vi "DefenderChute.vi"(6 "Current State":dbl=1.0, 7 "IA State Input 2":T1, 9 "balls":T5[](array[typedef])=[{"x"=-974.5169677734375, "y"=-3444.3310546875, "timestamp"=timestamp(2082759045.994995 s since 1904-01-01), "Vel_x"=0.0, "Vel_y"=0.0}], 10 "Field Size in":T6={"line_width"=10, "field_length"=9000, "field_width"=6000, "boundary_width"=250, "referee_width"=425, "goal_width"=700, "goal_depth"=180, "goal_wall_width"=20, "center_circle_radius"=500, "defense_radius"=500, "defense_stretch"=350, "free_kick_from_defense_dist"=700, "penalty_spot_from_field_line_dist"=450, "penalty_line_from_spot_dist"=350}, 11 "Robot in":T2={"id"=5, "function"=enum."Attacker", "x"=-983.1382446289062, "y"=-3000.010498046875, "orientation"=-1.5516623258590698, "v_tangent"=0.0, "v_normal"=0.0, "v_ang"=0.0, "kick_x"=0.0, "kick_z"=0.0, "dribble"=FALSE, "Timestamp"=timestamp(2082759045.994995 s since 1904-01-01), "dest_x"=0.0, "dest_y"=0.0, "dest_orientation"=0.0, "estimatives"={"est_v_tangent"=0.0, "est_v_normal"=0.0, "est_vx"=0.0, "est_vy"=0.0}, "dest_x_kick"=0.0, "dest_y_kick"=0.0, "Gap Coord"=[], "States"=enum."GoToTangent"}) -> (1 "Next State":dbl=1.0, 3 "Robot out":T2={"id"=5, "function"=enum."Attacker", "x"=-983.1382446289062, "y"=-3000.010498046875, "orientation"=-1.5516623258590698, "v_tangent"=0.0001540345015520423, "v_normal"=0.008599927144915481, "v_ang"=0.002668461263266586, "kick_x"=0.0, "kick_z"=0.0, "dribble"=FALSE, "Timestamp"=timestamp(2082759045.994995 s since 1904-01-01), "dest_x"=0.0, "dest_y"=0.0, "dest_orientation"=0.0, "estimatives"={"est_v_tangent"=0.0, "est_v_normal"=0.0, "est_vx"=0.0, "est_vy"=0.0}, "dest_x_kick"=0.0, "dest_y_kick"=0.0, "Gap Coord"=[], "States"=enum."GoToTangent"})   [LabVIEW 2016]
uses:
  Core/AI Robot.ctl
  Functions Enum.ctl
  AttackerStates.ctl
  Core/Field Size.ctl
  Core/AI Ball.ctl
  Core/AI Input.ctl
  Core/AI Judge.ctl
  Command Enum.ctl
  <vilib>/Analysis/coordinate.llb/2D Cartesian Coordinate Rotation (Scalar).vi
  <vilib>/Analysis/NI_AALPro.lvlib
panel:
  in  "Dist a frente da bola 2":dbl=150.0 format="%#_13g"
  in  "reckon timer":dbl=1.0 caption="Time Target (s)"
  out "Elapsed Time (s) 2":dbl caption="Elapsed Time (s)"
  out "Waveform Chart":dbl(graph)
  out "Elapsed Time (s)":dbl
  in  "Time Target \nto transition":dbl=0.5 caption="Time Target (s)"
  in  "Longe":dbl=300.0 format="%#_13g"
  in  "Cone de chute":dbl=0.09 format="%#_13g"
  in  "Perto":dbl=300.0 format="%#_13g"
  in  "Cone de rotação":dbl=1.1 format="%#_13g"
  in  "attacker farback":dbl=1500.0 format="%#_13g"
  in  "min dist to kick":dbl=150.0 format="%#_13g"
  in  "Dist a frente da bola":dbl format="%#_13g"
  in  "Constante do Renault":dbl=0.05
  in  "raio da circunferencia":dbl=175.0 format="%#_13g"
  in  "distance between ball and robot":dbl=275.0 format="%#_13g"
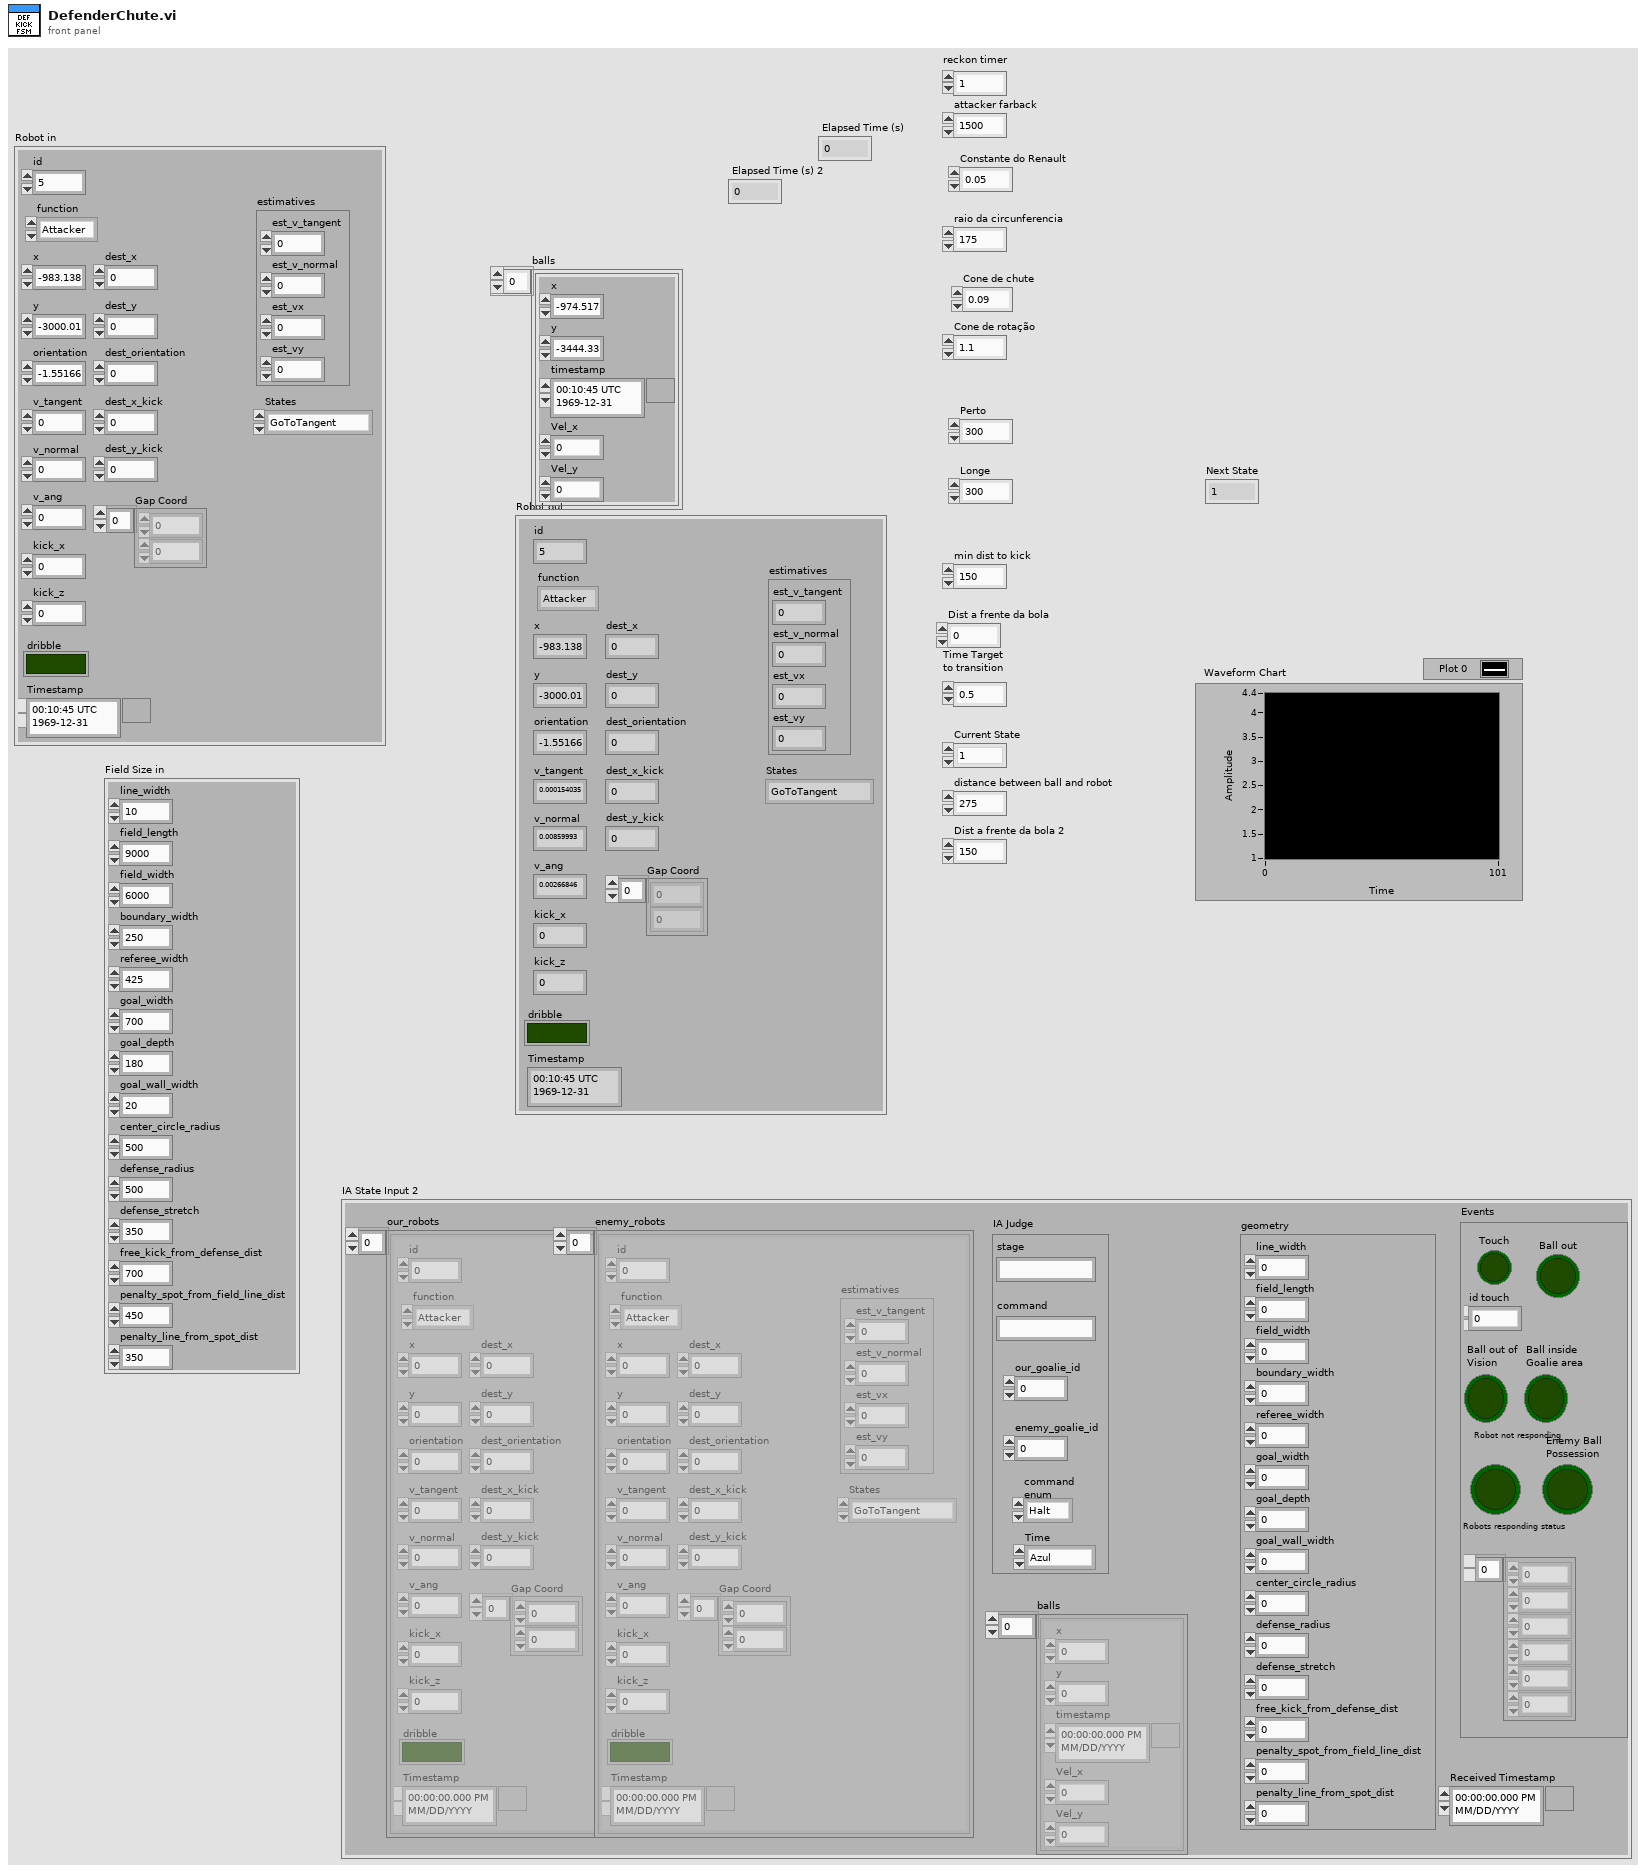
[diagram p1: front panel]
types:
  T1 = typedef "AI Input.ctl" = cluster{"our_robots":T2[], "enemy_robots":T2[], "balls":T5[], "geometry":T6, "IA Judge":T7, "Received Timestamp":timestamp, "Events":cluster{"Touch":bool, "Ball out":bool, "id touch":dbl, "Ball out of \nVision":bool, "Ball inside \nGoalie area":bool, "Robot not responding":bool, "Robots responding status":dbl[], "Enemy Ball \nPossession":bool}}
  T2 = typedef "AI Robot.ctl" = cluster{"id":u32, "function":T3, "x":dbl, "y":dbl, "orientation":dbl, "v_tangent":dbl, "v_normal":dbl, "v_ang":dbl, "kick_x":dbl, "kick_z":dbl, "dribble":bool, "Timestamp":timestamp, "dest_x":dbl, "dest_y":dbl, "dest_orientation":dbl, "estimatives":cluster{"est_v_tangent":dbl, "est_v_normal":dbl, "est_vx":dbl, "est_vy":dbl}, "dest_x_kick":dbl, "dest_y_kick":dbl, "Gap Coord":dbl[], "States":T4}
  T3 = typedef "Functions Enum.ctl" = enum16{"Attacker", "Goalie", "Defender", "Striker", "Goto 0", "Dummy", "Kicker", "ZigZag"}
  T4 = typedef "AttackerStates.ctl" = enum16{"Pass", "GoToTangent", "BallGetting", "GoToKick", ""}
  T5 = typedef "AI Ball.ctl" = cluster{"x":dbl, "y":dbl, "timestamp":timestamp, "Vel_x":dbl, "Vel_y":dbl}
  T6 = typedef "Field Size.ctl" = cluster{"line_width":u32, "field_length":u32, "field_width":u32, "boundary_width":u32, "referee_width":u32, "goal_width":u32, "goal_depth":u32, "goal_wall_width":u32, "center_circle_radius":u32, "defense_radius":u32, "defense_stretch":u32, "free_kick_from_defense_dist":u32, "penalty_spot_from_field_line_dist":u32, "penalty_line_from_spot_dist":u32}
  T7 = typedef "AI Judge.ctl" = cluster{"stage":string, "command":string, "our_goalie_id":dbl, "enemy_goalie_id":dbl, "command\nenum":T8, "Time":enum16{"Azul", "Amarelo"}}
  T8 = typedef "Command Enum.ctl" = enum16{"Halt", "Stop", "Force Start", "PKA Normal Start", "Prepare Kickoff Ally", "PKE Normal Start", "Prepare Kickoff Enemy", "Prepare Penalty Ally", "PPA Normal Start", "Prepare Penalty Enemy", "PPE Normal Start", "Direct Free Enemy", "Direct Free Ally", "Indirect Free Enemy", "Indirect Free Ally", "Timeout Enemy", "Timeout Ally", "Goal Enemy", "Goal Ally", "Ball Placement Enemy", "Ball Placement Ally", "None"}
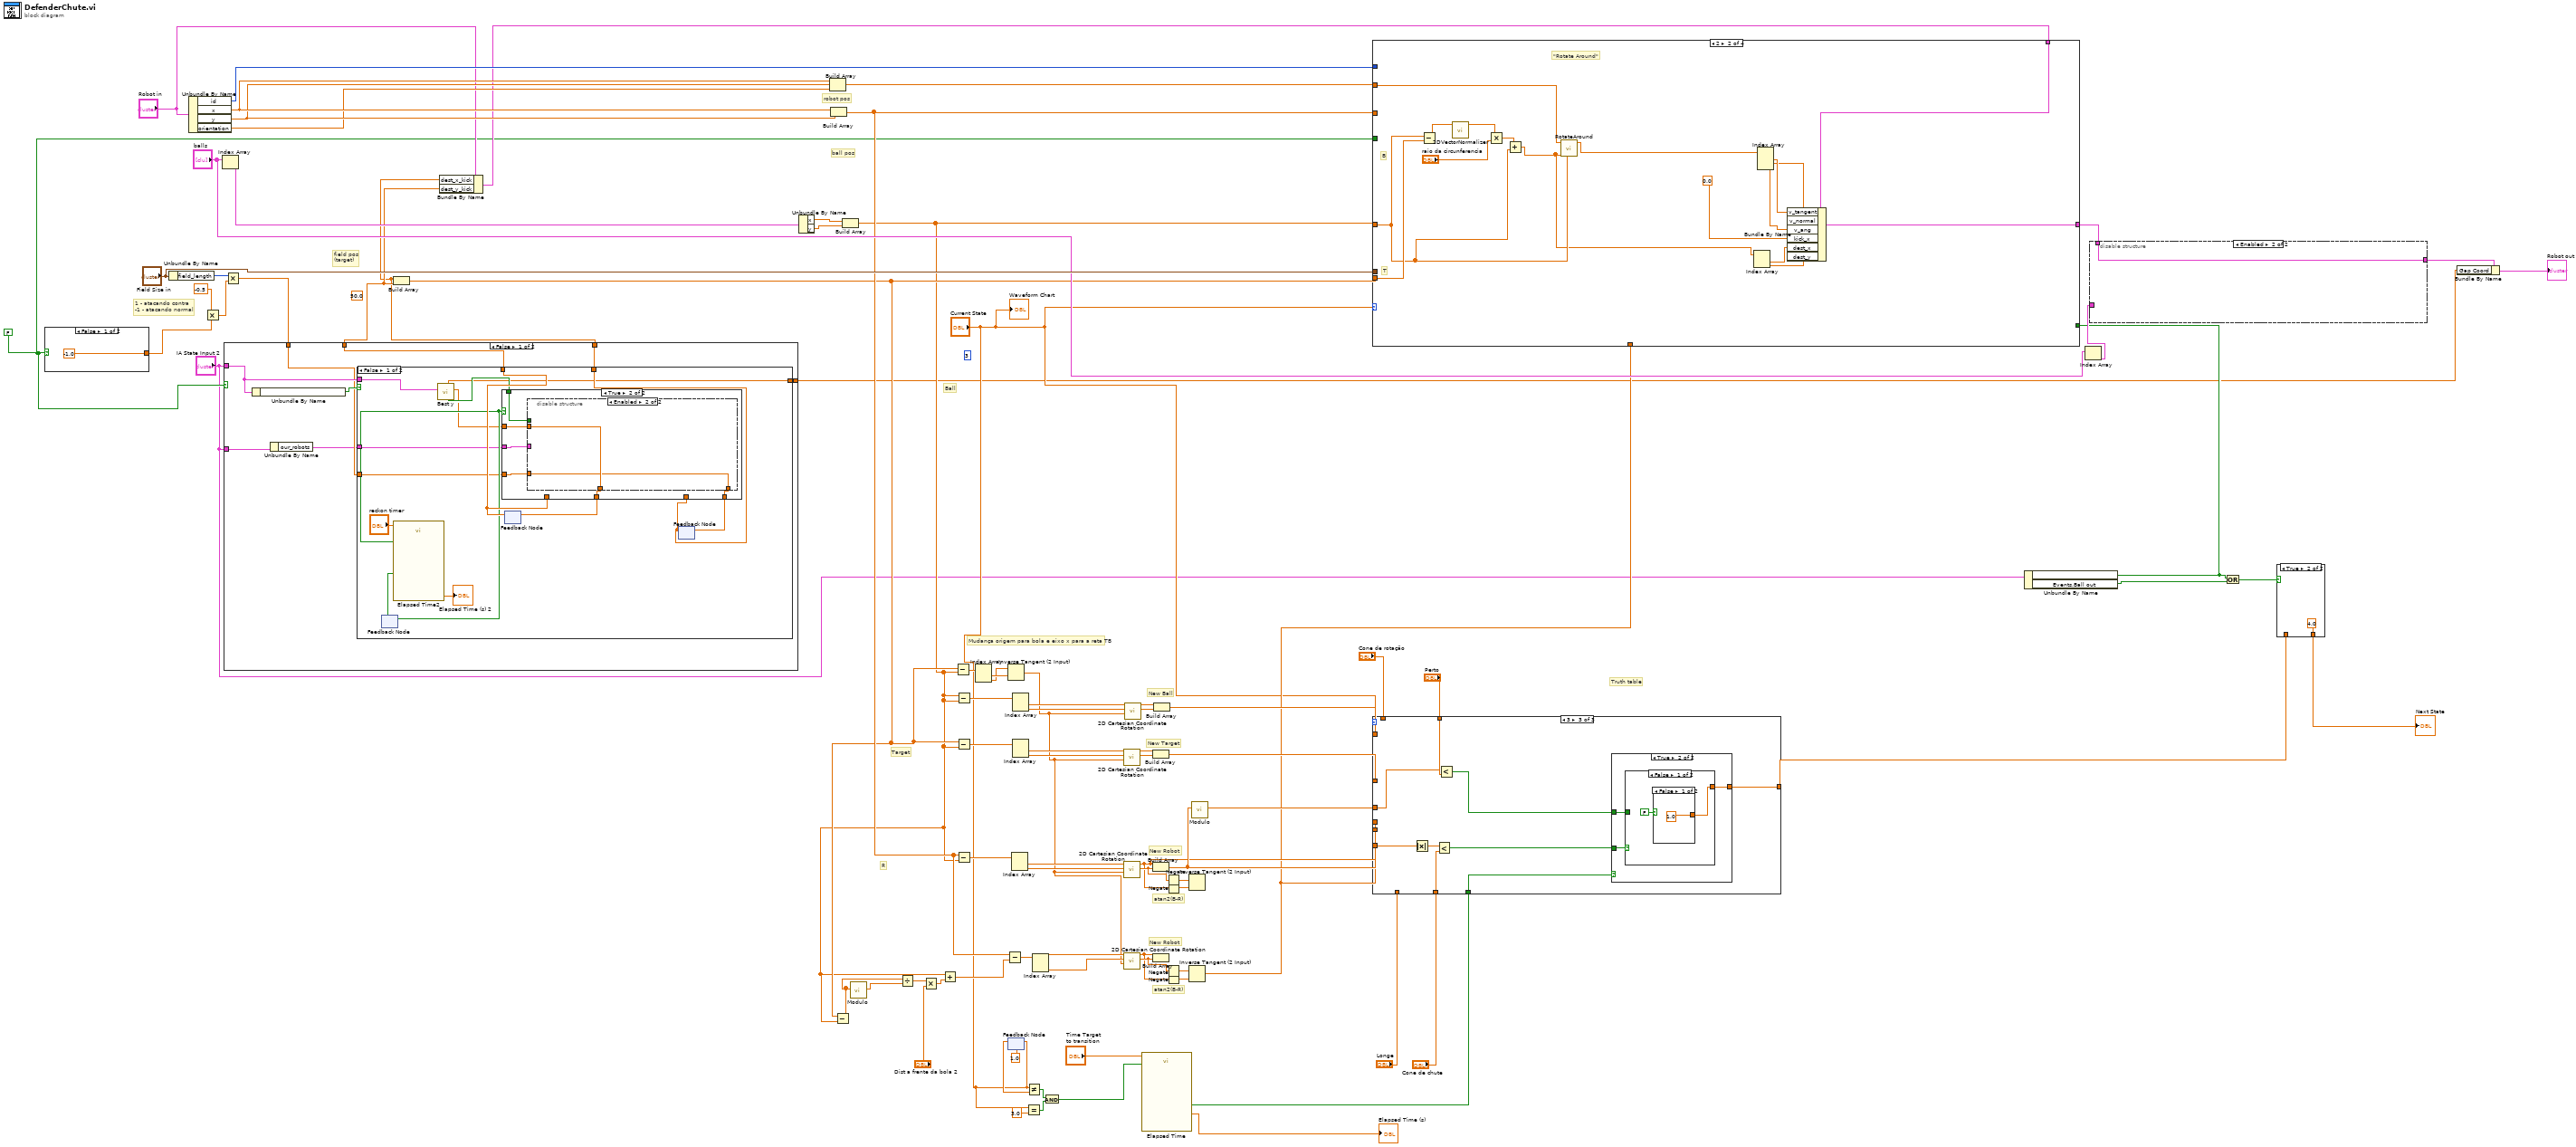
[diagram p0: block diagram]
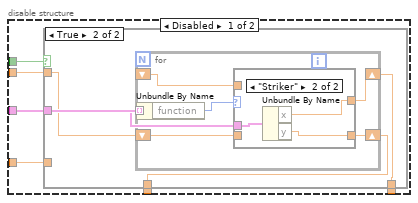
[diagram p3: hidden frame]
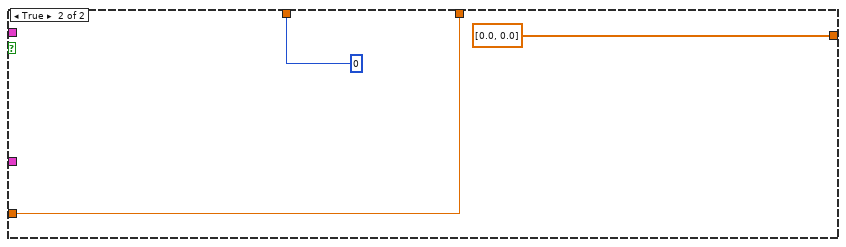
[diagram p6: hidden frame]
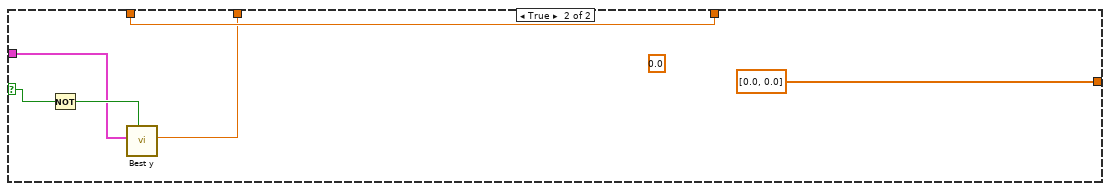
[diagram p7: hidden frame]
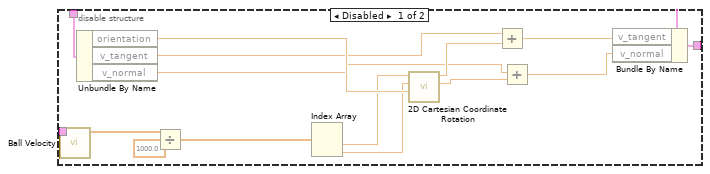
[diagram p8: hidden frame]
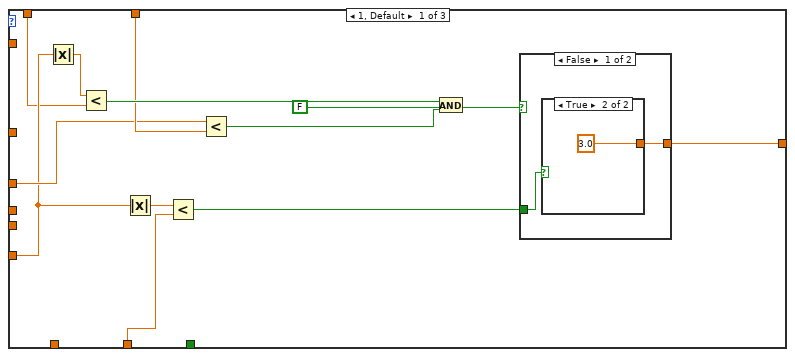
[diagram p9: hidden frame]
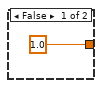
[diagram p10: hidden frame]
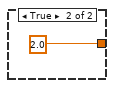
[diagram p11: hidden frame]
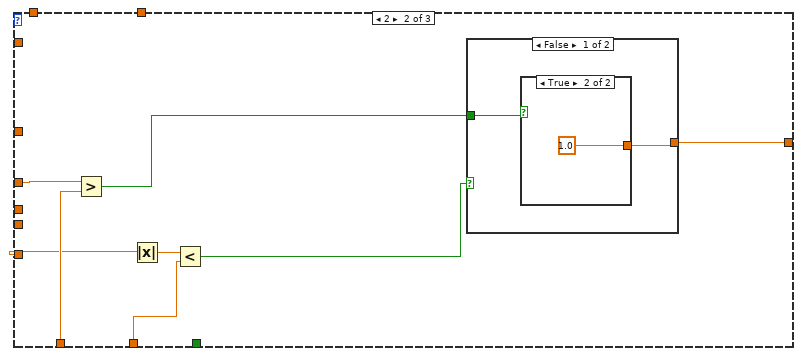
[diagram p12: hidden frame]
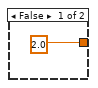
[diagram p13: hidden frame]
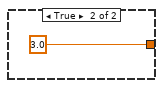
[diagram p14: hidden frame]
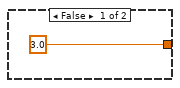
[diagram p15: hidden frame]
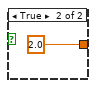
[diagram p16: hidden frame]
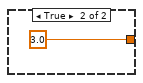
[diagram p17: hidden frame]
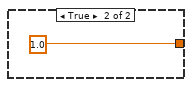
[diagram p19: hidden frame]
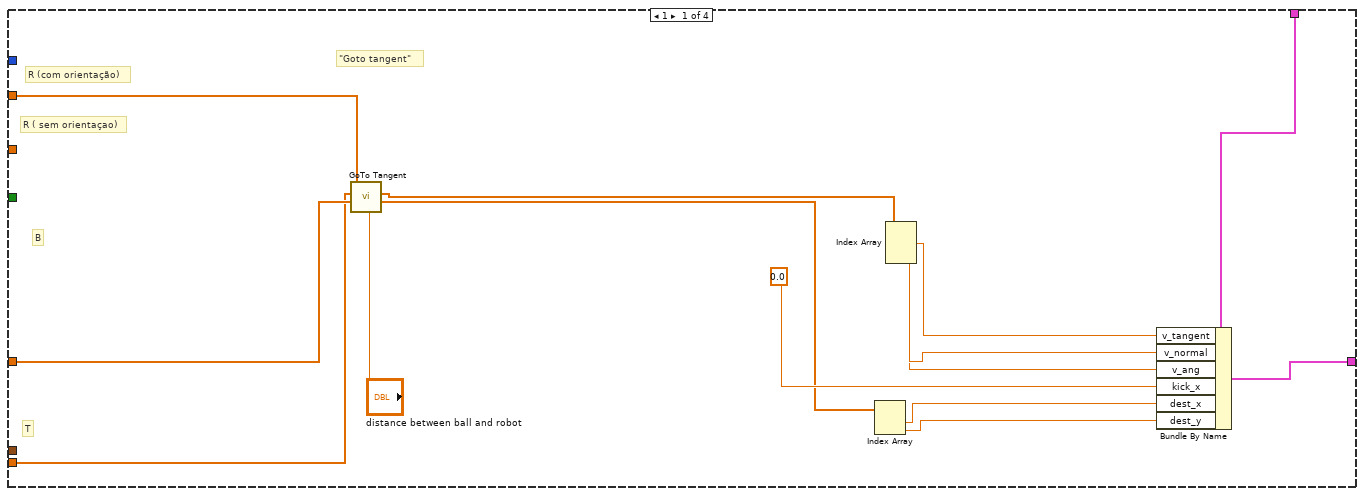
[diagram p20: hidden frame]
diagram:
  w8 = FALSE ("atacando contra?")
  (unwired) 50.0 ("element")
  (unwired) 3
  # "atan2(B-R)"
  # "New Robot"
  # "atan2(B-R)"
  # "New Robot"
  # "New Target"
  # "New Ball"
  # "R"
  # "Ball"
  # "Target"
  # "Mudança origem para bola e eixo x para a reta TB"
  # "1 - atacando contra\n-1 - atacando normal"
  # "Truth table"
  # "robot pos"
  # "field pos\n(target)"
  # "ball pos"
  n1 = case shown="False" w8 {
    tunnel: [-1.0 ("attck contra? 2") 1.0] -> w53
    frame False {
    }
    frame True {
    }
  }
  n2 = Unbundle By Name("Field Size in") -> ("field_length"=w86:u32)
  n3 = Unbundle By Name("Robot in") -> ("id"=w47:u32, "x"=w83:dbl, "y"=w82:dbl, "orientation"=w80:dbl)
  n4 = Multiply(x=-0.5, y=w53) -> (x*y=w78:dbl)
  n5 = Index Array(array="balls") -> (element=w87:T5)  [unwired: 1 in]
  n6 = Multiply(x=w86, y=w78) -> (x*y=w3:dbl)
  n7 = case shown="False" w8 {
    selector: w8 -> [_ w151]
    tunnel: "IA State Input 2" -> [w95 w149]
    tunnel: [w96 w148] -> w7
    tunnel: [w94 dbl[] [0.0, 0.0] ("Gap Coord")] -> w5
    tunnel: w3 -> [w93 w152]
    tunnel: [w92 w152] -> w2
    tunnel: "IA State Input 2" -> [w91 _]
    frame False {
      n8 = Unbundle By Name(w95) -> ("Events.Ball inside \nGoalie area"=w97:bool)
      n9 = Unbundle By Name(w91) -> ("our_robots"=w90:T2[])
      n10 = case shown="False" w97 {
        tunnel: [w109 0] -> w96
        tunnel: w95 -> [w111 _]
        tunnel: [w98 dbl[] [0.0, 0.0] ("Gap Coord")] -> w94
        tunnel: w93 -> [w102 w145]
        tunnel: [w101 w145] -> w92
        tunnel: w90 -> [w104 _]
        frame False {
          n11 = feedback #1() -> (w105:bool)  [unwired: 1 in]
          n12 = call "Elapsed Time2"("Time Target (s)"="reckon timer", "Auto Reset"=w105) -> ("Elapsed Time (s)"=→"Elapsed Time (s) 2":dbl, "Time has Elapsed"=w106:bool)  [unwired: 10 in, 6 out]
          n13 = feedback-in #1(w106) -> ()
          n14 = call "Best y.vi"("IA State"=w111) -> ("Best y"=w99:dbl, "Eclipse"=w100:bool, "Gap Coord"=w98:dbl[])  [unwired: 7 in, 1 out]
          n15 = feedback #2() -> (w109:dbl)  [unwired: 1 in]
          n16 = feedback #3() -> (w101:dbl)  [unwired: 1 in]
          n17 = case shown="True" w105 {
            tunnel: w99 -> [_ w118]
            tunnel: [w113 w119] -> w110
            tunnel: w109 -> [w113 _]
            tunnel: w100 -> [_ w117]
            tunnel: w104 -> [_ w116]
            tunnel: [w112 w115] -> w103
            tunnel: w102 -> [_ w114]
            tunnel: w101 -> [w112 _]
            frame False {
            }
            frame True {
              n18 = disable-structure shown="Enabled" {
                disable-tunnel: [w125 w144] -> w119
                disable-tunnel: w118 -> [w124 w144]
                disable-tunnel: w117 -> [w123 _]
                disable-tunnel: w116 -> [w122 _]
                disable-tunnel: [w121 w143] -> w115
                disable-tunnel: w114 -> [w120 w143]
                frame Disabled {
                  n19 = case shown="True" w123 {
                    tunnel: [w127 w130] -> w125
                    tunnel: w124 -> [w127 w129]
                    tunnel: w122 -> [_ w131]
                    tunnel: [w126 w128] -> w121
                    tunnel: w120 -> [w126 _]
                    frame False {
                    }
                    frame True {
                      n20 = for {
                        tunnel: w131 -> [w136] mode=indexing
                        shift-right: [w135] -> w128
                        shift-left: _ -> [w134]
                        shift-right: [w133] -> w130
                        shift-left: w129 -> [w132]
                        n21 = Unbundle By Name(w136) -> ("function"=w137:T3)
                        n22 = case shown="\"Striker\"" w137 {
                          tunnel: w136 -> [_ w142]
                          tunnel: [w138 w140] -> w135
                          tunnel: w134 -> [w138 _]
                          tunnel: [w139 w141] -> w133
                          tunnel: w132 -> [w139 _]
                          frame Default {
                          }
                          frame "Striker" {
                            n23 = Unbundle By Name(w142) -> ("x"=w140:dbl, "y"=w141:dbl)
                          }
                        }
                      }
                    }
                  }
                }
                frame Enabled {
                }
              }
            }
          }
          n24 = feedback-in #2(w110) -> ()
          n25 = feedback-in #3(w103) -> ()
        }
        frame True {
        }
      }
    }
    frame True {
      (unwired) 0.0 ("element")
      n26 = Not(x=w151) -> (.not. x?=w150:bool)
      n27 = call "Best y.vi"("inimigos"=w150, "IA State"=w149) -> ("Best y"=w148:dbl)  [unwired: 6 in, 3 out]
    }
  }
  n28 = Build Array(w2, w7) -> (w20:dbl[])
  n29 = Bundle By Name(cluster="Robot in", "dest_x_kick"=w2, "dest_y_kick"=w7) -> (w9:T2)
  n30 = Unbundle By Name(w87) -> ("x"=w85:dbl, "y"=w84:dbl)
  n31 = Build Array(w83, w82, w80) -> (w81:dbl[])
  n32 = Build Array(w83, w82) -> (w25:dbl[])
  n33 = Build Array(w85, w84) -> (w19:dbl[])
  n34 = Subtract(x=w20, y=w19) -> (x-y=w18:dbl[])
  n35 = call "Modulo.vi"("2D vector"=w18) -> ("Modulo"=w21:dbl)  [unwired: 10 in]
  n36 = Divide(x=w18, y=w21) -> (x/y=w22:dbl[])
  n37 = Multiply(x=w22, y="Dist a frente da bola 2") -> (x*y=w24:dbl[])
  n38 = Add(x=w19, y=w24) -> (x+y=w17:dbl[])
  n39 = Subtract(x=w20, y=w19) -> (x-y=w68:dbl[])
  n40 = Subtract(x=w19, y=w19) -> (x-y=w75:dbl[])
  n41 = Subtract(x=w20, y=w19) -> (x-y=w72:dbl[])
  n42 = Subtract(x=w25, y=w19) -> (x-y=w69:dbl[])
  n43 = Index Array(array=w68) -> (element #1=w67:dbl, element #2=w66:dbl)  [unwired: 2 in]
  n44 = Subtract(x=w25, y=w17) -> (x-y=w16:dbl[])
  n45 = Inverse Tangent (2 Input)(1:w67, 2:w66) -> (0:w13:dbl)
  n46 = feedback #4(1.0 ("Current State")) -> (w39:dbl)
  n47 = feedback-in #4("Current State") -> ()
  n48 = Index Array(array=w69) -> (element #1=w71:dbl, element #2=w70:dbl)  [unwired: 2 in]
  n49 = Index Array(array=w72) -> (element #1=w74:dbl, element #2=w73:dbl)  [unwired: 2 in]
  n50 = Index Array(array=w75) -> (element #1=w77:dbl, element #2=w76:dbl)  [unwired: 2 in]
  n51 = Equal?(x="Current State", y=3.0) -> (x = y?=w43:bool)
  n52 = Not Equal?(x="Current State", y=w39) -> (x != y?=w42:bool)
  n53 = Index Array(array=w16) -> (element #1=w15:dbl, element #2=w14:dbl)  [unwired: 2 in]
  n54 = And(x=w42, y=w43) -> (x .and. y?=w37:bool)
  n55 = call-poly <vilib>:"2D Cartesian Coordinate Rotation.vi"("theta"=w13, "y"=w70, "x"=w71) -> ("y out"=w50:dbl, "x out"=w49:dbl)  [unwired: 6 in, 1 out]
  n56 = call-poly <vilib>:"2D Cartesian Coordinate Rotation.vi"("theta"=w13, "y"=w14, "x"=w15) -> ("y out"=w27:dbl, "x out"=w26:dbl)  [unwired: 6 in, 1 out]
  n57 = call-poly <vilib>:"2D Cartesian Coordinate Rotation.vi"("theta"=w13, "y"=w73, "x"=w74) -> ("y out"=w64:dbl, "x out"=w65:dbl)  [unwired: 6 in, 1 out]
  n58 = call-poly <vilib>:"2D Cartesian Coordinate Rotation.vi"("theta"=w13, "y"=w76, "x"=w77) -> ("y out"=w62:dbl, "x out"=w63:dbl)  [unwired: 6 in, 1 out]
  n59 = call "Elapsed Time"("Time Target (s)"="Time Target \nto transition", "Reset"=w37) -> ("Elapsed Time (s)"=→"Elapsed Time (s)":dbl, "Time has Elapsed"=w45:bool)  [unwired: 10 in, 6 out]
  n60 = Build Array(w49, w50) -> (w57:dbl[])
  n61 = Build Array(w26, w27) -> ()  [unwired: 1 out]
  n62 = Build Array(w65, w64) -> (w58:dbl[])
  n63 = Build Array(w63, w62) -> (w59:dbl[])
  n64 = Negate(x=w50) -> (-x=w52:dbl)
  n65 = Negate(x=w49) -> (-x=w51:dbl)
  n66 = Negate(x=w27) -> (-x=w29:dbl)
  n67 = Negate(x=w26) -> (-x=w28:dbl)
  n68 = Inverse Tangent (2 Input)(1:w51, 2:w52) -> ()  [unwired: 1 out]
  n69 = Inverse Tangent (2 Input)(1:w28, 2:w29) -> (0:w12:dbl)
  n70 = call "Modulo.vi"("2D vector"=w57) -> ("Modulo"=w56:dbl)  [unwired: 10 in]
  n71 = case shown="3" "Current State" {
    tunnel: "Longe" -> [_ w177 _]
    tunnel: "Cone de chute" -> [w159 w172 w187]
    tunnel: w59 -> [_ _ _]
    tunnel: w58 -> [_ _ _]
    tunnel: w57 -> [_ _ _]
    tunnel: w56 -> [w162 w178 w190]
    tunnel: w12 -> [w157 w173 w188]
    tunnel: [w161 w176 w192] -> w55
    tunnel: "Perto" -> [w163 _ w191]
    tunnel: w49 -> [_ _ _]
    tunnel: w45 -> [_ _ w184]
    tunnel: "Cone de rotação" -> [w155 _ _]
    frame 1, Default {
      n72 = Absolute Value(x=w157) -> (abs(x)=w156:dbl)
      n73 = Less?(x=w156, y=w155) -> (x < y?=w165:bool)
      n74 = Absolute Value(x=w157) -> (abs(x)=w160:dbl)
      n75 = Less?(x=w160, y=w159) -> (x < y?=w158:bool)
      n76 = Less?(x=w162, y=w163) -> (x < y?=w164:bool)
      n77 = And(x=w165, y=w164) -> ()  [unwired: 1 out]
      n78 = case shown="False" FALSE {
        tunnel: [w167 2.0] -> w161
        tunnel: w158 -> [w166 _]
        frame False {
          n79 = case shown="True" w166 {
            tunnel: [1.0 3.0] -> w167
            frame False {
            }
            frame True {
            }
          }
        }
        frame True {
        }
      }
    }
    frame 2 {
      n80 = Greater?(x=w178, y=w177) -> (0:w175:bool)
      n81 = Absolute Value(x=w173) -> (abs(x)=w174:dbl)
      n82 = Less?(x=w174, y=w172) -> (x < y?=w171:bool)
      n83 = case shown="False" w171 {
        tunnel: [w179 3.0] -> w176
        tunnel: w175 -> [w180 _]
        frame False {
          n84 = case shown="True" w180 {
            tunnel: [2.0 1.0] -> w179
            frame False {
            }
            frame True {
            }
          }
        }
        frame True {
        }
      }
    }
    frame 3 {
      n85 = Absolute Value(x=w188) -> (abs(x)=w189:dbl)
      n86 = Less?(x=w189, y=w187) -> (x < y?=w186:bool)
      n87 = Less?(x=w190, y=w191) -> (x < y?=w185:bool)
      n88 = case shown="True" w184 {
        tunnel: [3.0 w196] -> w192
        tunnel: w186 -> [_ w195]
        tunnel: w185 -> [_ w194]
        frame False {
        }
        frame True {
          n89 = case shown="False" w195 {
            tunnel: [w198 3.0] -> w196
            tunnel: w194 -> [_ _]
            frame False {
              n90 = case shown="False" FALSE {
                tunnel: [1.0 2.0] -> w198
                frame False {
                }
                frame True {
                }
              }
            }
            frame True {
            }
          }
        }
      }
    }
  }
  n91 = Unbundle By Name("IA State Input 2") -> ("Events.Ball inside \nGoalie area"=w30:bool, "Events.Ball out"=w32:bool)
  n92 = case shown="2" "Current State" {
    tunnel: [w215 w232 w266 w284] -> w35
    tunnel: w9 -> [w214 w220 w265 w283]
    tunnel: w81 -> [w212 w231 w253 w275]
    tunnel: w25 -> [_ _ w240 w277]
    tunnel: w19 -> [w208 w219 w244 w278]
    tunnel: w20 -> [w207 w225 w258 _]
    tunnel: "Field Size in" -> [_ _ _ w276]
    tunnel: w47 -> [_ _ _ _]
    tunnel: w30 -> [_ _ _ w270]
    tunnel: w8 -> [_ _ _ w269]
    tunnel: w12 -> [_ _ w236 _]
    frame 1 {
      # "\"Goto tangent\""
      # "B"
      # "T"
      # "R ( sem orientaçao)"
      # "R (com orientação)"
      n93 = call "GoTo Tangent.vi"("distance between ball and robot"="distance between ball and robot", "Ball"=w208, "Target"=w207, "R"=w212) -> ("Destination"=w204:dbl[], "Output\nVelocity"=w206:dbl[])  [unwired: 6 in]
      n94 = Index Array(array=w204) -> (element #1=w203:dbl, element #2=w202:dbl)  [unwired: 2 in]
      n95 = Index Array(array=w206) -> (element #1=w211:dbl, element #2=w210:dbl, element #3=w209:dbl)  [unwired: 3 in]
      n96 = Bundle By Name(cluster=w214, "v_tangent"=w211, "v_normal"=w210, "v_ang"=w209, "kick_x"=0.0, "dest_x"=w203, "dest_y"=w202) -> (w215:T2)
    }
    frame 2 {
      # "T"
      # "B"
      # "\"Rotate Around\""
      n97 = Subtract(x=w219, y=w225) -> (x-y=w224:dbl[])
      n98 = call "2DVectorNormalizer.vi"("2D vector"=w224) -> ("2D vector 2"=w223:dbl[])  [unwired: 10 in]
      n99 = Multiply(x=w223, y="raio da circunferencia") -> (x*y=w221:dbl[])
      n100 = Add(x=w221, y=w219) -> (x+y=w218:dbl[])
      n101 = call "RotateAround.vi"("Centre"=w219, "Target"=w218, "Position"=w231) -> ("Output\nVelocity"=w226:dbl[])  [unwired: 8 in]
      n102 = Index Array(array=w218) -> (element #1=w217:dbl, element #2=w216:dbl)  [unwired: 2 in]
      n103 = Index Array(array=w226) -> (element #1=w229:dbl, element #2=w228:dbl, element #3=w227:dbl)  [unwired: 3 in]
      n104 = Bundle By Name(cluster=w220, "v_tangent"=w229, "v_normal"=w228, "v_ang"=w227, "kick_x"=0.0, "dest_x"=w217, "dest_y"=w216) -> (w232:T2)
    }
    frame 3 {
      # "BT"
      # "ball-target angle"
      # "B"
      # "T"
      # "R ( sem orientaçao)"
      # "R (com orientação)"
      # "\"Goto and kick\""
      n105 = Subtract(x=w258, y=w240) -> (x-y=w245:dbl[])
      n106 = call "Modulo.vi"("2D vector"=w245) -> ("Modulo"=w246:dbl)  [unwired: 10 in]
      n107 = Index Array(array=w245) -> (element #1=w260:dbl, element #2=w259:dbl)  [unwired: 2 in]
      n108 = Inverse Tangent (2 Input)(1:w260, 2:w259) -> (0:w257:dbl)
      n109 = Divide(x=w245, y=w246) -> (x/y=w247:dbl[])
      n110 = Multiply(x=w247, y="Dist a frente da bola") -> (x*y=w250:dbl[])
      n111 = Add(x=w244, y=w250) -> (x+y=w248:dbl[])
      n112 = Index Array(array=w248) -> (element #1=w256:dbl, element #2=w255:dbl)  [unwired: 2 in]
      n113 = Build Array(w256, w255, w257) -> (w242:dbl[])
      n114 = call "distance.vi"("target pos"=w244, "obj pos"=w240) -> ("sqrt(x)"=w264:dbl)  [unwired: 9 in]
      n115 = call "GoTo.vi"("Target"=w242, "Position"=w253) -> ("Output\nVelocity"=w254:dbl[])  [unwired: 8 in, 1 out]
      n116 = Less?(x=w264, y="min dist to kick") -> (x < y?=w262:bool)
      n117 = Index Array(array=w242) -> (element #1=w243:dbl, element #2=w241:dbl)  [unwired: 2 in]
      n118 = Index Array(array=w254) -> (element #1=w252:dbl, element #2=w239:dbl, element #3=w251:dbl)  [unwired: 3 in]
      n119 = Subtract(x=w236, y=3.14) -> (x-y=w234:dbl)
      n120 = Multiply(x="Constante do Renault", y=w234) -> (x*y=w237:dbl)
      n121 = Add(x=w239, y=w237) -> (x+y=w238:dbl)
      n122 = case shown="True" w262 {
        tunnel: [0.0 5.0] -> w263
        frame False {
        }
        frame True {
        }
      }
      n123 = Bundle By Name(cluster=w265, "dest_x"=w243, "dest_y"=w241, "v_tangent"=w252, "v_normal"=w238, "v_ang"=w251, "kick_x"=w263) -> (w266:T2)
    }
    frame Default {
      n124 = case shown="True" w270 {
        tunnel: w278 -> [w288 w300]
        tunnel: w277 -> [w287 w297]
        tunnel: w276 -> [w286 w299]
        tunnel: [w285 w305] -> w273
        tunnel: w269 -> [_ w293]
        frame False {
          n125 = call "PosBolaFora.vi"("Field Size in"=w286, "Position da bola"=w288, "Position do robot"=w287) -> ("Target"=w285:dbl[])  [unwired: 8 in]
        }
        frame True {
          # "ball-target angle"
          n126 = Unbundle By Name(w299) -> ("field_length"=w296:u32)
          n127 = Subtract(x=w300, y=w297) -> (x-y=w303:dbl[])
          n128 = Index Array(array=w300) -> (element #1=w292:dbl, element #2=w306:dbl)  [unwired: 2 in]
          n129 = Index Array(array=w303) -> (element #1=w301:dbl, element #2=w302:dbl)  [unwired: 2 in]
          n130 = Divide(x=w296, y=u32 2) -> (x/y=w294:dbl)
          n131 = Subtract(x=w294, y="attacker farback") -> (x-y=w291:dbl)
          n132 = Sign(1:w292) -> (0:w290:dbl)
          n133 = Multiply(x=w291, y=w290) -> (x*y=w289:dbl)
          n134 = Inverse Tangent (2 Input)(1:w301, 2:w302) -> ()  [unwired: 1 out]
          n135 = case shown="True" w293 {
            tunnel: w289 -> [w307 w310]
            tunnel: [w307 w309] -> w304
            frame False {
            }
            frame True {
              n136 = Multiply(x=w310, y=-1.0) -> (x*y=w309:dbl)
            }
          }
          n137 = Build Array(w304, w306) -> (w305:dbl[])
        }
      }
      n138 = call "GoTo.vi"("Target"=w273, "Position"=w275) -> ("Output\nVelocity"=w274:dbl[])  [unwired: 8 in, 1 out]
      n139 = Index Array(array=w274) -> (element #1=w281:dbl, element #2=w280:dbl, element #3=w279:dbl)  [unwired: 3 in]
      n140 = Index Array(array=w273) -> (element #1=w272:dbl, element #2=w271:dbl)  [unwired: 2 in]
      n141 = Bundle By Name(cluster=w283, "v_tangent"=w281, "v_normal"=w280, "v_ang"=w279, "kick_x"=0.0, "dest_x"=w272, "dest_y"=w271) -> (w284:T2)
    }
  }
  n142 = Index Array(array="balls") -> (element=w34:T5)  [unwired: 1 in]
  n143 = disable-structure shown="Enabled" {
    disable-tunnel: w35 -> [w318 w326]
    disable-tunnel: [w315 w326] -> w6
    disable-tunnel: w34 -> [w314 _]
    frame Disabled {
      n144 = call "Ball Velocity.vi"("Ball"=w314) -> ("Velocity"=w312:dbl[])  [unwired: 10 in]
      n145 = Unbundle By Name(w318) -> ("orientation"=w325:dbl, "v_tangent"=w321:dbl, "v_normal"=w319:dbl)
      n146 = Divide(x=w312, y=1000.0) -> (x/y=w313:dbl[])
      n147 = Index Array(array=w313) -> (element #1=w323:dbl, element #2=w324:dbl)  [unwired: 2 in]
      n148 = call-poly <vilib>:"2D Cartesian Coordinate Rotation.vi"("theta"=w325, "y"=w324, "x"=w323) -> ("y out"=w320:dbl, "x out"=w322:dbl)  [unwired: 6 in, 1 out]
      n149 = Add(x=w321, y=w322) -> (x+y=w317:dbl)
      n150 = Add(x=w319, y=w320) -> (x+y=w316:dbl)
      n151 = Bundle By Name(cluster=w318, "v_tangent"=w317, "v_normal"=w316) -> (w315:T2)
    }
    frame Enabled {
    }
  }
  n152 = Or(x=w30, y=w32) -> (x .or. y?=w31:bool)
  n153 = case shown="True" w31 {
    tunnel: [w327 4.0] -> w40
    tunnel: w55 -> [w327 _]
    frame False {
    }
    frame True {
    }
  }
  "Next State" <- w40
  n154 = Bundle By Name(cluster=w6, "Gap Coord"=w5) -> (→"Robot out":T2)
  "Waveform Chart" <- "Current State"
